vi "Convert to Two Byte.vi"(7 "Input Method (0:String)":u16(ring) items=["String", "Number"], 9 "Input Number":i32, 10 "Numeric String":string="1000") -> (2 "Output String":string)   [LabVIEW 2015, in "SDG X Series.lvlib"]
doc: "Converts an ASCII numeric string to a 2-byte hexadecimal string in little endian order."
uses:
  <instrlib>/SDG X Series/SDG X Series.lvlib
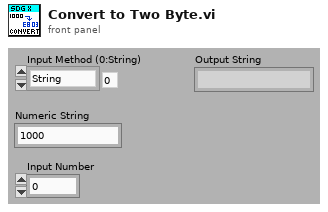
[diagram p1: front panel]
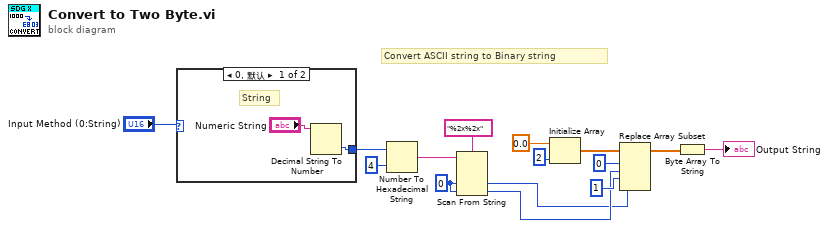
[diagram p0: block diagram]
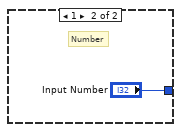
[diagram p2: hidden frame]
diagram:
  w11 = 0 ("default value 1")
  # "Convert ASCII string to Binary string"
  n1 = case shown="0, 默认" "Input Method (0:String)" {
    tunnel: [w17 "Input Number"] -> w12
    frame 0, Default {
      # "String"
      n2 = Decimal String To Number(string="Numeric String") -> (number=w17:i32)  [unwired: 2 in, 1 out]
    }
    frame 1 {
      # "Number"
    }
  }
  n3 = Number To Hexadecimal String(1:i16 4 ("width (-)"), 2:w12) -> (0:w14:string)
  n4 = Scan From String(format string="%2x%2x", input string=w14, default 1=w11, default 2=w11) -> (output 1=w2:i32, output 2=w3:i32)  [unwired: 2 in, 3 out]
  n5 = Initialize Array(0.0 ("element"), 2) -> (w9:dbl[])
  n6 = Replace Array Subset(array=w9, new element #1=w3, index #1=0, new element #2=w2, index #2=1) -> (w6:dbl[])
  n7 = Byte Array To String(unsigned byte array=w6) -> (string=→"Output String":string)
